vi "X.vi"   [LabVIEW 2016]
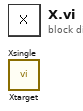
[diagram p0: block diagram]
diagram:
  n1 = call "Xtarget.vi"() -> ()  [unwired: 9 in, 1 out]
  n2 = call "Xsingle.vi"() -> ()  [unwired: 9 in, 1 out]
